vi "get device information.vi"(8 "error in (no error)":errorcluster, 10 "device_information":T1, 11 "id":i32) -> (0 "error out":errorcluster, 2 "device_information out":T1, 3 "function return":i32)   [LabVIEW 2012, in "libximc.lvlib"]
doc: "result_t XIMC_API get_device_information (device_t id, device_information_t* device_information);"
uses:
  libximc.lvlib
  libximc.dll
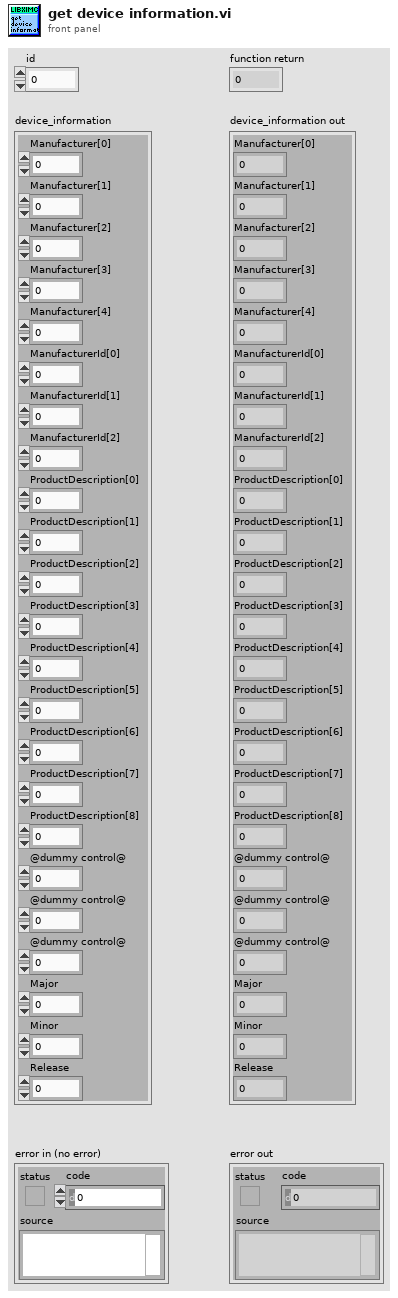
[diagram p1: front panel]
types:
  T1 = cluster{"Manufacturer[0]":i8, "Manufacturer[1]":i8, "Manufacturer[2]":i8, "Manufacturer[3]":i8, "Manufacturer[4]":i8, "ManufacturerId[0]":i8, "ManufacturerId[1]":i8, "ManufacturerId[2]":i8, "ProductDescription[0]":i8, "ProductDescription[1]":i8, "ProductDescription[2]":i8, "ProductDescription[3]":i8, "ProductDescription[4]":i8, "ProductDescription[5]":i8, "ProductDescription[6]":i8, "ProductDescription[7]":i8, "ProductDescription[8]":i8, "@dummy control@":i8, "@dummy control@":i8, "@dummy control@":i8, "Major":u32, "Minor":u32, "Release":u32}
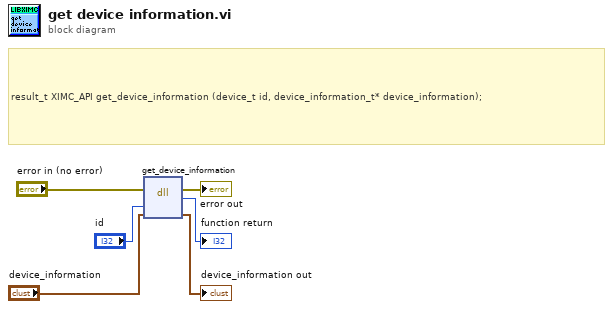
[diagram p0: block diagram]
diagram:
  # "result_t XIMC_API get_device_information (device_t id, device_information_t* device_information);"
  n1 = dll-call lib="C:/Users/Vasily/Att_examples/LabVIEW_example/libximc.*" fn="get_device_information"(error in="error in (no error)", "id"="id", "device_information"="device_information") -> (error out=→"error out":errorcluster, →"function return":i32, "device_information"=→"device_information out":T1)  [unwired: 3 in, 1 out]
